vi "XLP80_EA_WriteOutputs_Rekuperation.vi"(8 "err in":errorcluster, 11 "Device information":string[](array[string])=["ASRL1::INSTR", "EL 3160-60 A", "000", "///", "1", "160", "60", "400", "10", "400"]) -> (0 "err out":errorcluster, 3 "Device information IN":string[](array[string])=["ASRL1::INSTR", "EL 3160-60 A", "000", "///", "1", "160", "60", "400", "10", "400"])   [LabVIEW 2021]
uses:
  XLP80_EA_Globals.vi
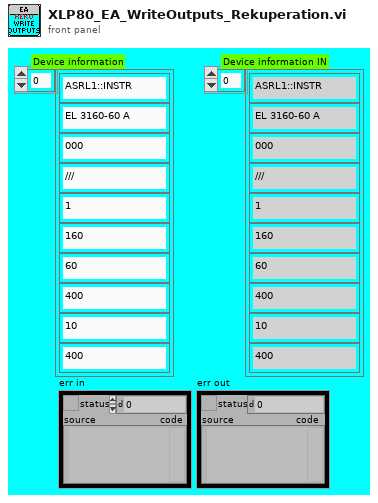
[diagram p1: front panel]
types:
  T1 = typedef "XLP80_EA_TDefsCluster_EA Setpoint_Reku.ctl" = cluster{"Load":bool, "Set Current":sgl, "Set Voltage":sgl, "Set Power":sgl}
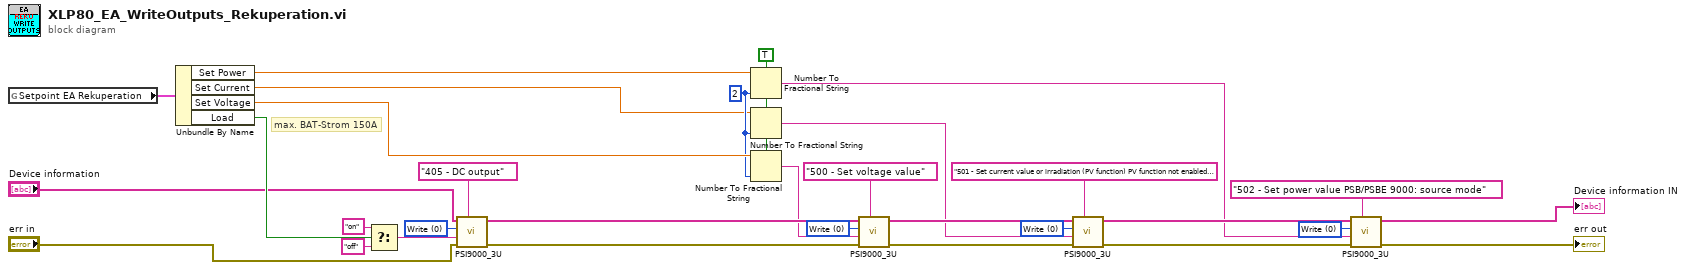
[diagram p0: block diagram]
diagram:
  w12 = u8 0 items=["Write", "Read"] ("Access")
  w16 = u8 0 items=["Write", "Read"] ("Access")
  w17 = u8 0 items=["Write", "Read"] ("Access")
  w7 = TRUE ("use system decimal point (T)")
  w6 = i16 2 ("precision (6)")
  w26 = u8 0 items=["Write", "Read"] ("Access")
  # "max. BAT-Strom 150A"
  n1 = global read "XLP80_EA_Globals.vi" "Setpoint EA Rekuperation"() -> (w31:T1)
  n2 = Unbundle By Name(w31) -> ("Set Power"=w8:sgl, "Set Current"=w2:sgl, "Set Voltage"=w27:sgl, "Load"=w30:bool)
  n3 = Select(t="on" ("Value"), s=w30, f="off") -> (s? t:f=w25:string)
  n4 = call <instrlib>:"PSI9000_3U.vi"("Command list"="405 - DC output", "Error in"="err in", "Value"=w25, "Access"=w26, "Device information in"="Device information") -> ("Error out"=w22:errorcluster, "Device information out"=w23:string[])  [unwired: 1 in, 2 out]
  n5 = Number To Fractional String(use system decimal point (T)=w7, number=w8, precision (6)=w6) -> (F-format string=w5:string)  [unwired: 1 in]
  n6 = Number To Fractional String(use system decimal point (T)=w7, number=w2, precision (6)=w6) -> (F-format string=w18:string)  [unwired: 1 in]
  n7 = Number To Fractional String(use system decimal point (T)=w7, number=w27, precision (6)=w6) -> (F-format string=w19:string)  [unwired: 1 in]
  n8 = call <instrlib>:"PSI9000_3U.vi"("Command list"="500 - Set voltage value", "Error in"=w22, "Value"=w19, "Access"=w17, "Device information in"=w23) -> ("Error out"=w21:errorcluster, "Device information out"=w20:string[])  [unwired: 1 in, 2 out]
  n9 = call <instrlib>:"PSI9000_3U.vi"("Command list"="501 - Set current value or irradiation (PV function) PV function not enabled for PSB/PSBEE PSB/PSBE 9000: source mode", "Error in"=w21, "Value"=w18, "Access"=w16, "Device information in"=w20) -> ("Error out"=w4:errorcluster, "Device information out"=w11:string[])  [unwired: 1 in, 2 out]
  n10 = call <instrlib>:"PSI9000_3U.vi"("Command list"="502 - Set power value PSB/PSBE 9000: source mode", "Error in"=w4, "Value"=w5, "Access"=w12, "Device information in"=w11) -> ("Error out"=→"err out":errorcluster, "Device information out"=→"Device information IN":string[])  [unwired: 1 in, 2 out]
